vi "Read serian-num.vi"(8 "error in (no error)":errorcluster, 11 "Product in":refnum<class "Product.lvclass">) -> (0 "error out":errorcluster, 2 "serian-num":dbl, 3 "Product out":refnum<class "Product.lvclass">)   [LabVIEW 2018, in "Product.lvclass"]
uses:
  Product.lvclass
  Product.lvclass/Product.ctl
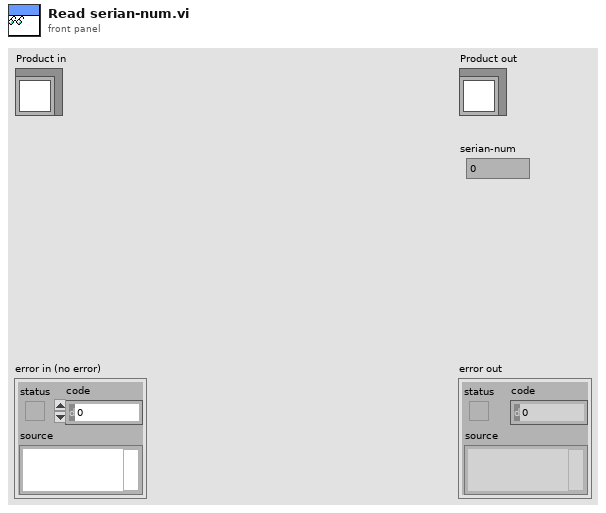
[diagram p1: front panel]
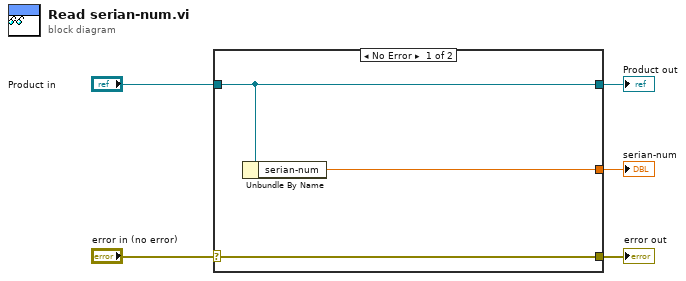
[diagram p0: block diagram]
diagram:
  n1 = case shown="No Error" "error in (no error)" {
    selector: "error in (no error)" -> [w8 w9]
    tunnel: [w8 w9] -> w4
    tunnel: [w7 w10] -> w2
    tunnel: "Product in" -> [w7 w10]
    tunnel: [w6 _] -> w1
    frame No Error {
      n2 = Unbundle By Name(w7) -> ("serian-num"=w6:dbl)
    }
    frame Error {
    }
  }
  "error out" <- w4
  "Product out" <- w2
  "serian-num" <- w1
